vi "备用系数写入.vi"(7 "备用系数":cluster{"上限":dbl, "下限":dbl, "范围":dbl}, 8 "error in (no error)":errorcluster caption="错误输入（无错误）", 9 "量程":enum16{"低量程", "高量程"}(ring), 10 "测量模式":T1(ring), 11 "测量参数":u16(ring) items=["总磷"=1, "总氮"=2, "氨氮"=3, "COD"=22]) -> (0 "error out":errorcluster caption="错误输出")   [LabVIEW 2016, in "斯坦道总氮.lvlib"]
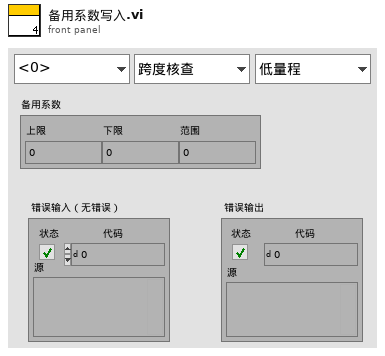
[diagram p1: front panel]
types:
  T1 = enum16{"跨度核查", "水样测量", "零点核查", "标样核查", "加标回收", "快捷测试", "空白校准", "标样校准"}
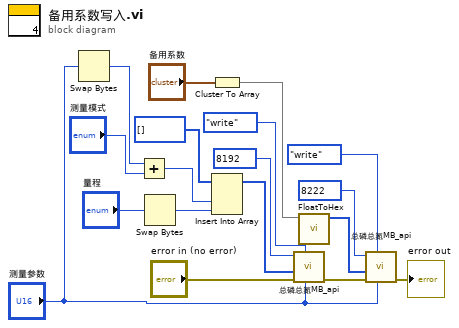
[diagram p0: block diagram]
diagram:
  n1 = Swap Bytes(anything="测量参数") -> (byte swapped=w4:u16)
  n2 = Add(x=w4, y="测量模式") -> (x+y=w13:u16)
  n3 = Swap Bytes(anything="量程") -> (byte swapped=w2:u16)
  n4 = Cluster To Array(cluster="备用系数") -> (array=w17:dbl[])
  n5 = Insert Into Array(array=u16[] [] ("数组"), new element #1=w13, new element #2=w2) -> (w7:u16[])  [unwired: 1 in]
  n6 = call "总磷总氮MB_api.vi"("Slave ID"="测量参数", "STEP"=enum16{"open", "read", "write", "close"}."write", "Error in"="error in (no error)", "values"=w7, "starting address"=u16 8192) -> ("error out"=w10:errorcluster)  [unwired: 4 in, 2 out]
  n7 = call "FloatToHex.vi"("浮点数"=w17) -> ("DCBA整形输出"=w6:u16[])  [unwired: 10 in]
  n8 = call "总磷总氮MB_api.vi"("Slave ID"="测量参数", "STEP"=enum16{"open", "read", "write", "close"}."write", "Error in"=w10, "values"=w6, "starting address"=u16 8222) -> ("error out"=→"error out":errorcluster)  [unwired: 4 in, 2 out]
